vi "CheckStatus.vi"(8 "error in (no error)":errorcluster, 11 "VISA resource name":refnum<visa-resource-name>) -> (0 "error out":errorcluster, 1 "Ques Status":u16, 2 "Oper Status":u16, 3 "VISA resource name out":refnum<visa-resource-name>, 4 "Ques Status bits":bool[](array[boolean]), 6 "Oper Status bits":bool[](array[boolean]))   [LabVIEW 2019, in "Tektronix AFG 3000 Series.lvlib"]
doc: "Enables or disables the output connector."
uses:
  <userlib>/Tektronix AFG 3000 Series/Tektronix AFG 3000 Series.lvlib
panel:
  out "Ques Status String":string
  out "Oper Status String":string
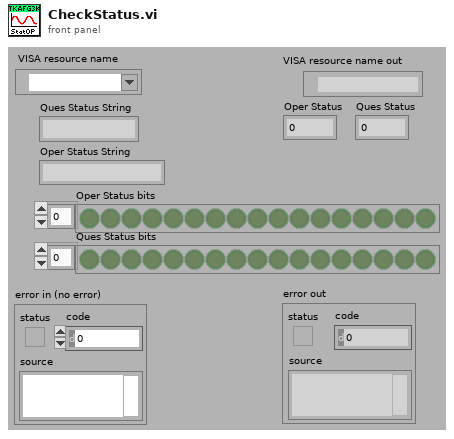
[diagram p1: front panel]
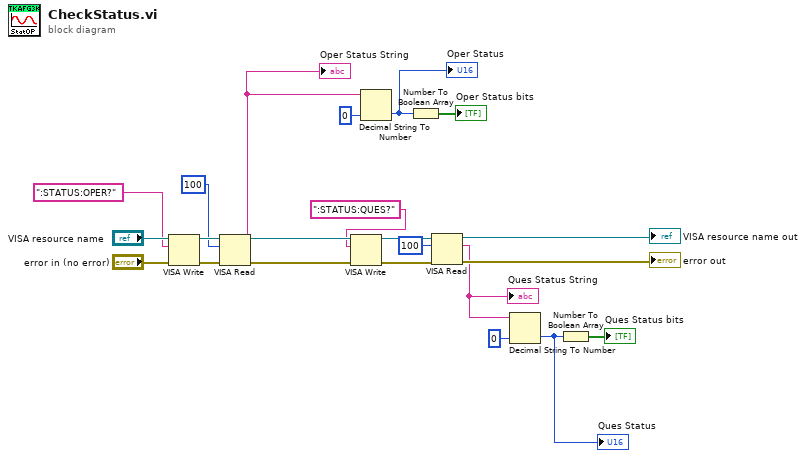
[diagram p0: block diagram]
diagram:
  n1 = VISA Write(VISA resource name="VISA resource name", write buffer=":STATUS:OPER?" ("string (\"\")"), error in (no error)="error in (no error)") -> (VISA resource name out=w19:refnum<visa-resource-name>, error out=w18:errorcluster)  [unwired: 1 out]
  n2 = VISA Read(VISA resource name=w19, byte count=u32 100 ("nombre d'octets"), error in (no error)=w18) -> (VISA resource name out=w11:refnum<visa-resource-name>, read buffer=w16:string, error out=w12:errorcluster)  [unwired: 1 out]
  "Oper Status String" <- w16
  n3 = VISA Write(VISA resource name=w11, write buffer=":STATUS:QUES?" ("string (\"\")"), error in (no error)=w12) -> (VISA resource name out=w8:refnum<visa-resource-name>, error out=w9:errorcluster)  [unwired: 1 out]
  n4 = Decimal String To Number(string=w16, default (0L)=u16 0 ("valeur par défaut (0 I32)")) -> (number=w15:u16)  [unwired: 1 in, 1 out]
  "Oper Status" <- w15
  n5 = Number To Boolean Array(number=w15) -> (Boolean array=→"Oper Status bits":bool[])
  n6 = VISA Read(VISA resource name=w8, byte count=u32 100 ("nombre d'octets"), error in (no error)=w9) -> (VISA resource name out=→"VISA resource name out":refnum<visa-resource-name>, read buffer=w2:string, error out=→"error out":errorcluster)  [unwired: 1 out]
  "Ques Status String" <- w2
  n7 = Decimal String To Number(string=w2, default (0L)=u16 0 ("valeur par défaut (0 I32)")) -> (number=w3:u16)  [unwired: 1 in, 1 out]
  "Ques Status" <- w3
  n8 = Number To Boolean Array(number=w3) -> (Boolean array=→"Ques Status bits":bool[])
